vi "S2C_5190CR_Proc_Measure.vi"(7 "Local?":bool, 8 "Error In":errorcluster, 10 "Command":string, 11 "JSON String":string) -> (0 "Error Out":errorcluster, 3 "Response":variant)   [LabVIEW 2015]
doc: "Measures either Current, Power, or Voltage for the selected outlet."
uses:
  S2C_5190CR_Proc_Globals.vi
  <vilib>/regexp/Match Regular Expression.xnode
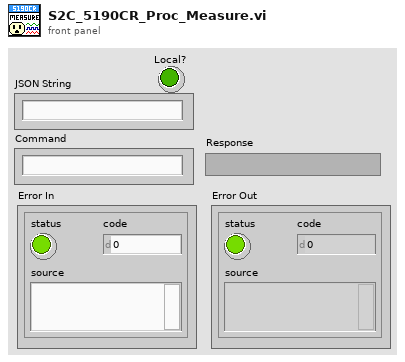
[diagram p1: front panel]
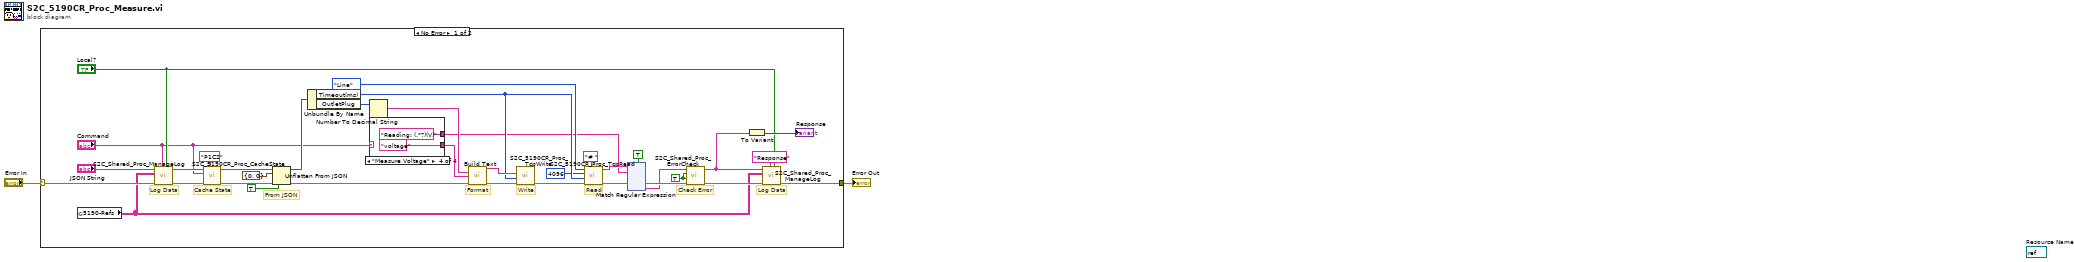
[diagram p0: block diagram]
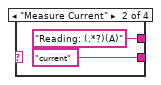
[diagram p3: hidden frame]
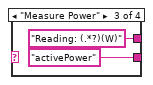
[diagram p4: hidden frame]
diagram:
  (unwired) refnum<visa-resource-name> refnum  # Resource Name
  n1 = case shown="No Error" "Error In" {
    selector: "Error In" -> [w36 w161]
    tunnel: [w27 w161] -> w1
    frame No Error {
      w3 = TRUE ("ExpReply?")
      # "Read"
      # "Check Error"
      # "Write"
      # "Format"
      # "Cache State"
      # "Log Data"
      # "Log Data"
      # "From JSON"
      n2 = global read "S2C_5190CR_Proc_Globals.vi" "5190-Refs"() -> (w17:string[][])
      n3 = call "S2C_Shared_Proc_ManageLog.vi"("Local?"="Local?", "Command"="Command", "Error In"=w36, "Refs"=w17, "Data In"="JSON String") -> ("Error Out"=w32:errorcluster, "Data Out"=w31:string)  [unwired: 5 in]
      n4 = call "S2C_5190CR_Proc_CacheState.vi"("Label"="P1C2", "Error In"=w32, "Command"="Command", "Data In"=w31) -> ("Error Out"=w29:errorcluster, "Data Out"=w30:string)  [unwired: 6 in]
      n5 = Unflatten From JSON(JSON string=w30, type and defaults=cluster{"OutletPlug":u16, "Timeout(ms)":i32} {"OutletPlug"=0, "Timeout(ms)"=0} ("P1C2"), default null elements? (F)=TRUE, error in (no error)=w29) -> (value=w26:cluster{"OutletPlug":u16, "Timeout(ms)":i32}, error out=w24:errorcluster)  [unwired: 3 in]
      n6 = Unbundle By Name(w26) -> ("Timeout(ms)"=w13:i32, "OutletPlug"=w25:u16)
      n7 = Number To Decimal String(number=w25) -> (decimal integer string=w23:string)  [unwired: 1 in]
      n8 = case shown="\"Measure Voltage\"" "Command" {
        tunnel: [_ "current" "activePower" "voltage"] -> w22
        tunnel: [_ "Reading: (.*?)(A)" ("regular expression") "Reading: (.*?)(W)" ("regular expression") "Reading: (.*?)(V)" ("regular expression")] -> w7
        frame "Other", Default {
        }
        frame "Measure Current" {
        }
        frame "Measure Power" {
        }
        frame "Measure Voltage" {
        }
      }
      n9 = call "Build Text"("Outlet"=w23, "Meas"=w22, "error in (no error)"=w24) -> ("Result"=w14:string, "error out"=w21:errorcluster)  [unwired: 11 in]
      n10 = call "S2C_5190CR_Proc_TcpWrite.vi"("Error In"=w21, "Timeout(ms)"=w13, "Data"=w14) -> ("Error Out"=w20:errorcluster)  [unwired: 8 in]
      n11 = call "S2C_5190CR_Proc_TcpRead.vi"("Line Seperator"="# " ("line separator"), "Error In"=w20, "Timeout(ms)"=w13, "Bytes"=4096, "Read Mode"=enum16{"Normal", "Line"}."Line" ("Write Mode")) -> ("Error Out"=w9:errorcluster, "Data"=w8:string)  [unwired: 5 in]
      n12 = xnode "Match Regular Expression"("input string"=w8, "regular expression"=w7, "error in"=w9, "multiline? (F)"=TRUE) -> ("error out"=w5:errorcluster, "submatch 1"=w4:string)  [unwired: 2 in, 4 out]
      n13 = call "S2C_Shared_Proc_ErrorCheck.vi"("Error In"=w5, "ExpReply?"=w3, "Clear Error?"=w3, "Reply Text"=w4) -> ("Error Out"=w19:errorcluster, "Status"=w18:string)  [unwired: 6 in]
      n14 = To Variant(anything=w18) -> (Variant=→"Response":variant)
      n15 = call "S2C_Shared_Proc_ManageLog.vi"("Local?"="Local?", "Command"="Response", "Error In"=w19, "Refs"=w17, "Data In"=w18) -> ("Error Out"=w27:errorcluster)  [unwired: 5 in, 1 out]
    }
    frame Error {
    }
  }
  "Error Out" <- w1
